vi "updateCategoryDefaultAmount.vi"(8 "error in (no error)":errorcluster, 10 "Category":refnum<class "Category.lvclass">, 11 "Account History in":refnum<class "Account History.lvclass">) -> (0 "error out":errorcluster, 3 "Account History out":refnum<class "Account History.lvclass">)   [LabVIEW 2018, in "Account History.lvclass"]
uses:
  Account History.lvclass
  Category/Category.lvclass
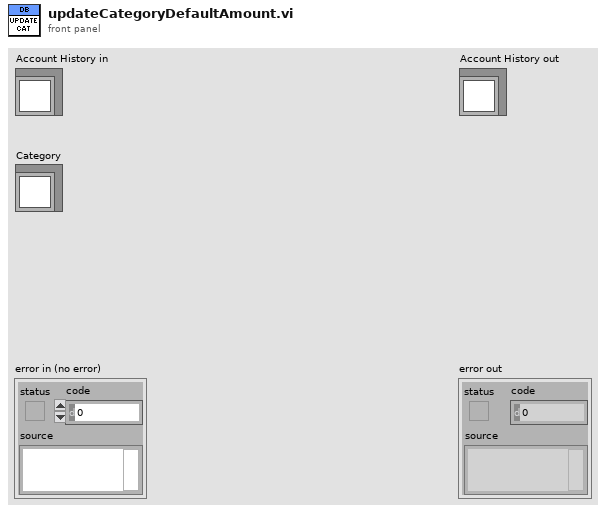
[diagram p1: front panel]
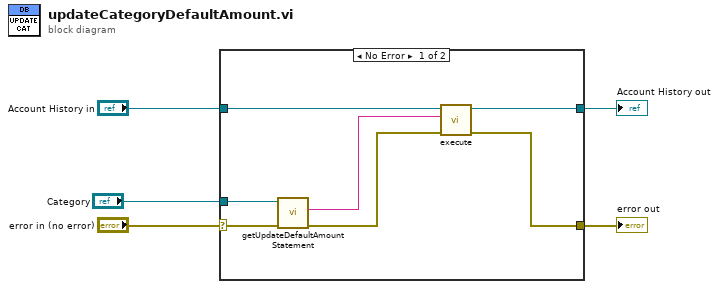
[diagram p0: block diagram]
diagram:
  n1 = case shown="No Error" "error in (no error)" {
    selector: "error in (no error)" -> [w11 w14]
    tunnel: [w6 w14] -> w4
    tunnel: [w8 w13] -> w2
    tunnel: "Account History in" -> [w10 w13]
    tunnel: "Category" -> [w12 _]
    frame No Error {
      n2 = call "getUpdateDefaultAmountStatement.vi"("error in (no error)"=w11, "Category in"=w12) -> ("error out"=w7:errorcluster, "Update Statement"=w9:string)  [unwired: 7 in, 1 out]
      n3 = call "execute.vi"("error in (no error)"=w7, "SQL query"=w9, "Database in"=w10) -> ("error out"=w6:errorcluster, "Database out"=w8:refnum<class "Account History.lvclass">)  [unwired: 7 in]
    }
    frame Error {
    }
  }
  "error out" <- w4
  "Account History out" <- w2
